vi "WiiCoords.vi"(11 "error in (no error)":errorcluster) -> (6 "X":i32, 8 "Y":i32, 13 "A":bool, 14 "Home":bool, 15 "error out":errorcluster)   [LabVIEW 2010]
uses:
  ola/Speaker Example/Action Engines/AE Access VIs/AE - Bluetooth ButtonAccData.vi
  ola/Speaker Example/Action Engines/AE Access VIs/AE - Bluetooth IRData.vi
panel:
  out "IR State":bool[](array[boolean])
  # "Press \"Home\" for STOP"
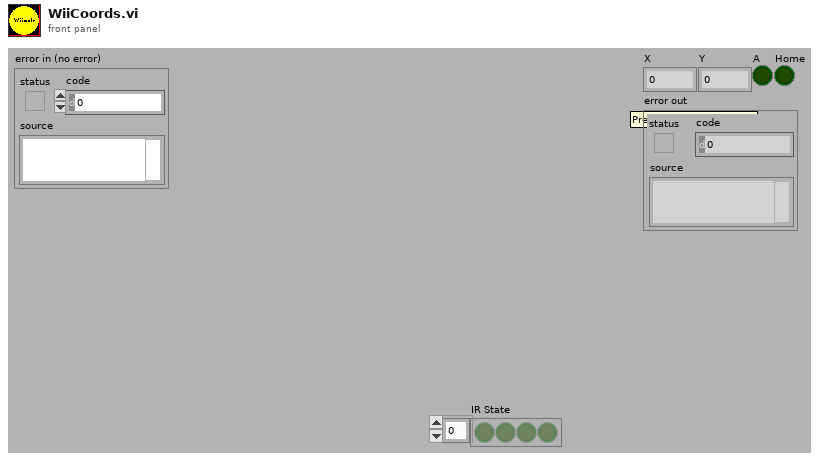
[diagram p1: front panel]
types:
  T1 = typedef "WiimoteState.ctl" = cluster{"X":sgl, "Y":sgl, "Z":sgl, "A":bool, "B":bool, "Down":bool, "Home":bool, "Left":bool, "Minus":bool, "One":bool, "Plus":bool, "Right":bool, "Two":bool, "Up":bool, "error out":errorcluster}
  T2 = typedef "WiimoteState(IR).ctl" = cluster{"Mode":u8, "IR State":bool[], "X Values":sgl[], "Y Values":sgl[], "Raw X Values":i32[], "Raw Y Values":i32[], "Sizes":i32[], "X Midpoint":sgl, "Y Midpoint":sgl}
  T3 = typedef "LVAllMonitorsDisplayTypeDef.ctl" = cluster{"Bounds":cluster{"Left":i16, "Top":i16, "Right":i16, "Bottom":i16}, "Depth":i16}[]
  T4 = cluster{"Bounds":cluster{"Left":i16, "Top":i16, "Right":i16, "Bottom":i16}, "Depth":i16}
  T5 = cluster{"Left":i16, "Top":i16, "Right":i16, "Bottom":i16}
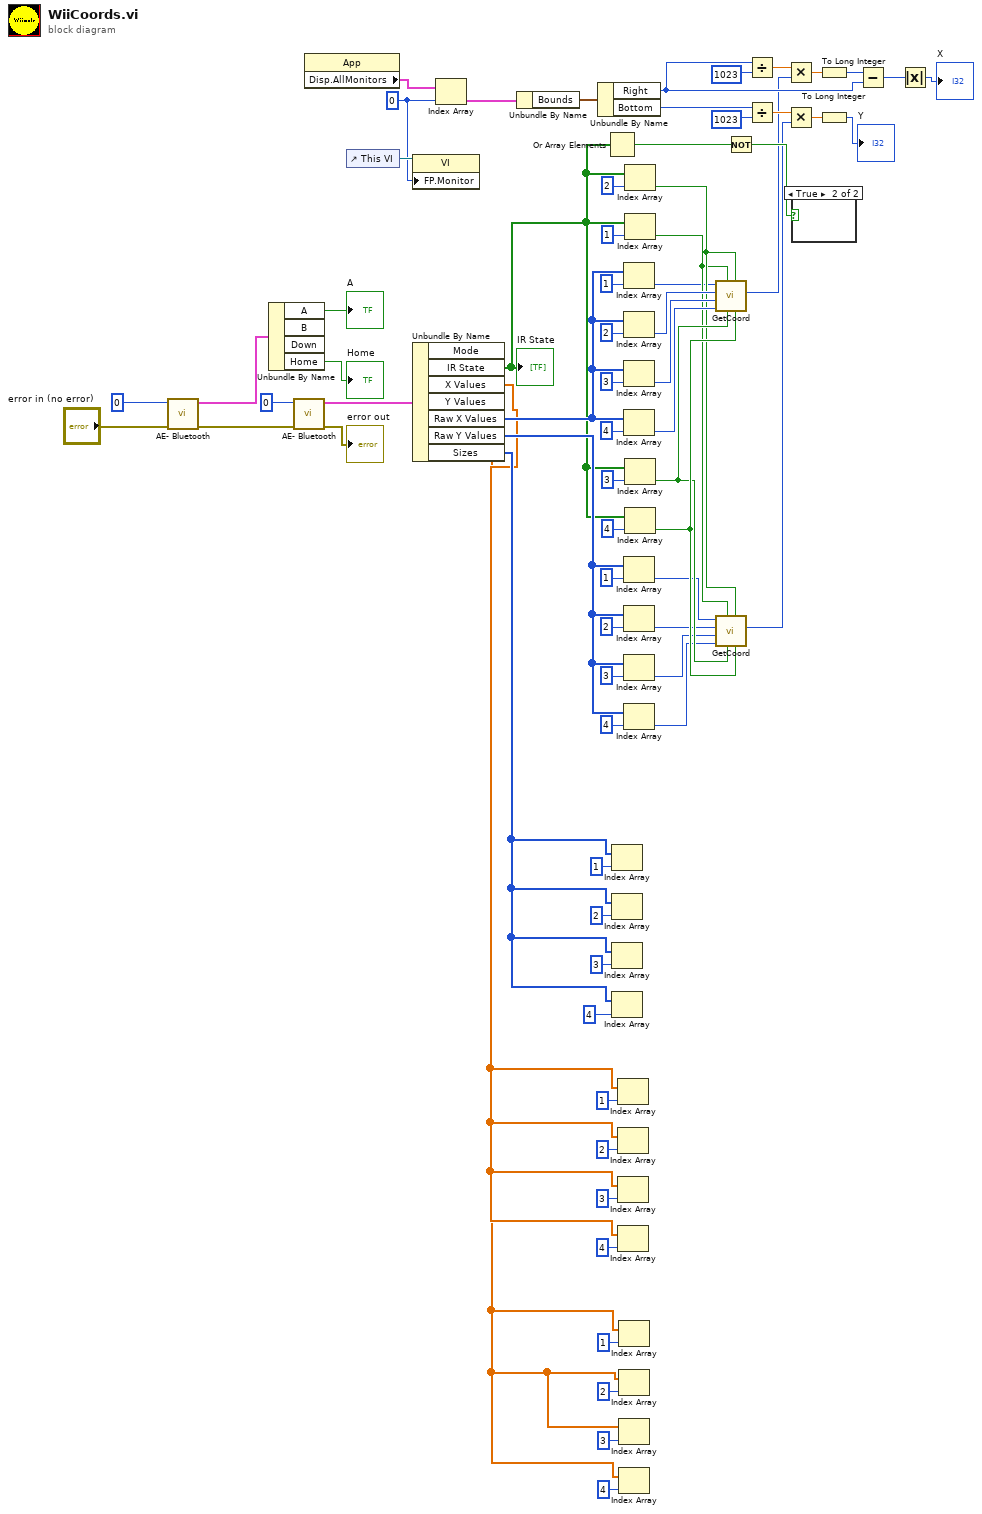
[diagram p0: block diagram]
diagram:
  w40 = u16 0 ("Front Panel Window:Monitor")
  n1 = call-poly "AE- Bluetooth.vi"("error in (no error)"="error in (no error)", "Wiimote"=0) -> ("error out"=w69:errorcluster, "Wiimote State"=w68:T1)  [unwired: 8 in]
  n2 = Unbundle By Name(w68) -> ("A"=→"A":bool, "Home"=→"Home":bool)  [unwired: 2 out]
  n3 = call-poly "AE- Bluetooth.vi"("error in (no error)"=w69, "Wiimote"=0) -> ("error out"=→"error out":errorcluster, "IRState"=w70:T2)  [unwired: 8 in]
  n4 = property class="App"() -> ("Disp.AllMonitors"=w39:T3)  [unwired: 2 in, 2 out]
  n5 = control-ref of="This VI"() -> (w42:refnum<vi>)
  n6 = property class="VI"(reference=w42, "FP.Monitor"=w40) -> ()  [unwired: 1 in, 2 out]
  n7 = Unbundle By Name(w70) -> ("IR State"=w29:bool[], "X Values"=w6:sgl[], "Y Values"=w1:sgl[], "Raw X Values"=w58:i32[], "Raw Y Values"=w53:i32[], "Sizes"=w15:i32[])  [unwired: 1 out]
  "IR State" <- w29
  n8 = Index Array(array=w39, index=w40) -> (element=w41:T4)
  n9 = Unbundle By Name(w41) -> ("Bounds"=w38:T5)
  n10 = Unbundle By Name(w38) -> ("Right"=w26:i16, "Bottom"=w25:i16)
  n11 = Or Array Elements(Boolean array=w29) -> (logical OR=w28:bool)
  n12 = Index Array(array=w15, index=1) -> ()  [unwired: 1 out]
  n13 = Index Array(array=w15, index=2) -> ()  [unwired: 1 out]
  n14 = Index Array(array=w15, index=3) -> ()  [unwired: 1 out]
  n15 = Index Array(array=w15, index=4) -> ()  [unwired: 1 out]
  n16 = Index Array(array=w6, index=1) -> ()  [unwired: 1 out]
  n17 = Index Array(array=w6, index=2) -> ()  [unwired: 1 out]
  n18 = Index Array(array=w6, index=3) -> ()  [unwired: 1 out]
  n19 = Index Array(array=w6, index=4) -> ()  [unwired: 1 out]
  n20 = Index Array(array=w1, index=1) -> ()  [unwired: 1 out]
  n21 = Index Array(array=w1, index=2) -> ()  [unwired: 1 out]
  n22 = Index Array(array=w1, index=3) -> ()  [unwired: 1 out]
  n23 = Index Array(array=w1, index=4) -> ()  [unwired: 1 out]
  n24 = Index Array(array=w58, index=1) -> (element=w19:i32)
  n25 = Index Array(array=w58, index=2) -> (element=w52:i32)
  n26 = Index Array(array=w58, index=3) -> (element=w51:i32)
  n27 = Index Array(array=w58, index=4) -> (element=w50:i32)
  n28 = Index Array(array=w53, index=1) -> (element=w18:i32)
  n29 = Index Array(array=w53, index=2) -> (element=w45:i32)
  n30 = Index Array(array=w53, index=3) -> (element=w44:i32)
  n31 = Index Array(array=w53, index=4) -> (element=w43:i32)
  n32 = Index Array(array=w29, index=2) -> (element=w47:bool)
  n33 = Index Array(array=w29, index=1) -> (element=w46:bool)
  n34 = Index Array(array=w29, index=3) -> (element=w48:bool)
  n35 = Index Array(array=w29, index=4) -> (element=w49:bool)
  n36 = call "GetCoord.vi"(4:"4"=w49, 5:"2"=w47, 6:"3"=w48, 7:"1"=w46, 8:"4"=w50, 9:"3"=w51, 10:"2"=w52, 11:"1"=w19) -> ("OUT"=w16:i32)  [unwired: 3 in]
  n37 = call "GetCoord.vi"(4:"4"=w49, 5:"2"=w47, 6:"3"=w48, 7:"1"=w46, 8:"4"=w43, 9:"3"=w44, 10:"2"=w45, 11:"1"=w18) -> ("OUT"=w17:i32)  [unwired: 3 in]
  n38 = Not(x=w28) -> (.not. x?=w27:bool)
  n39 = Divide(x=w26, y=i16 1023) -> (x/y=w36:dbl)
  n40 = Divide(x=w25, y=i16 1023) -> (x/y=w33:dbl)
  n41 = Multiply(x=w36, y=w16) -> (x*y=w35:dbl)
  n42 = Multiply(x=w33, y=w17) -> (x*y=w32:dbl)
  n43 = case shown="True" w27 {
    frame False {
    }
    frame True {
    }
  }
  n44 = To Long Integer(number=w35) -> (32bit integer=w31:i32)
  n45 = To Long Integer(number=w32) -> (32bit integer=→"Y":i32)
  n46 = Subtract(x=w31, y=w26) -> (x-y=w30:i32)
  n47 = Absolute Value(x=w30) -> (abs(x)=→"X":i32)
